vi "LStrPrintf.vi"(8 "error in (no error)":errorcluster, 10 "ObjectPointer":i64) -> (0 "error out":errorcluster, 2 "OutputStr":string)   [LabVIEW 2022 SP3, in "openDAQ.lvlib" / "daqUtils.lvlib"]
uses:
  daqUtils.lvlib
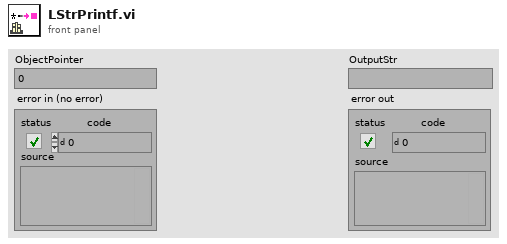
[diagram p1: front panel]
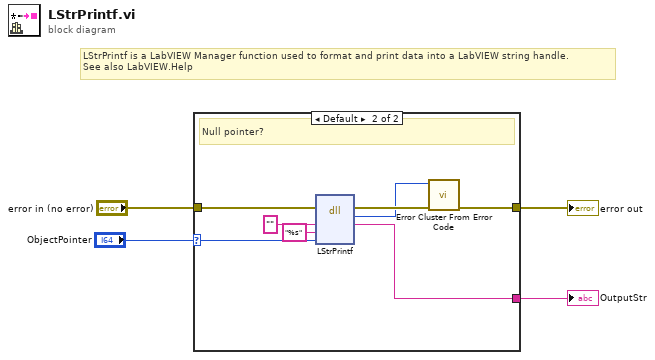
[diagram p0: block diagram]
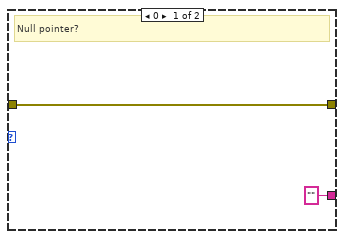
[diagram p2: hidden frame]
diagram:
  # "LStrPrintf is a LabVIEW Manager function used to format and print data into a LabVIEW string handle.\nSee also LabVIEW.Help"
  n1 = case shown="Default" "ObjectPointer" {
    selector: "ObjectPointer" -> [_ w7]
    tunnel: "error in (no error)" -> [w6 w10]
    tunnel: ["" ("string") w9] -> w3
    tunnel: [w6 w8] -> w2
    frame 0 {
      # "Null pointer?"
    }
    frame Default {
      # "Null pointer?"
      n2 = dll-call lib="LabVIEW" fn="LStrPrintf"(error in=w10, "string"="", "format"="%s", "arg"=w7) -> (error out=w12:errorcluster, "return type"=w11:i32, "string"=w9:string)  [unwired: 4 in, 1 out]
      n3 = call <vilib>:"Error Cluster From Error Code.vi"("error in (no error)"=w12, "error code (0)"=w11) -> ("error out"=w8:errorcluster)  [unwired: 7 in]
    }
  }
  "OutputStr" <- w3
  "error out" <- w2
